vi "Set Visibility Of Queue List.vi"(8 "error in (no error)":errorcluster, 10 "Visible":bool, 11 "SongQueueActor in":refnum<class "SongQueueActor.lvclass">) -> (0 "error out":errorcluster, 3 "SongQueueActor out":refnum<class "SongQueueActor.lvclass">)   [LabVIEW 2015, in "SongQueueActor.lvlib" / "SongQueueActor.lvclass"]
uses:
  SongQueueActor.lvclass
  SongQueueActor.lvclass/SongQueueActor.ctl
  builds/xctls/Song Queue/Song Queue.lvlibp/app/xctls/SongQueue/Song Queue.xctl
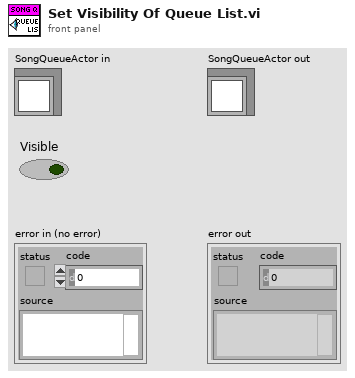
[diagram p1: front panel]
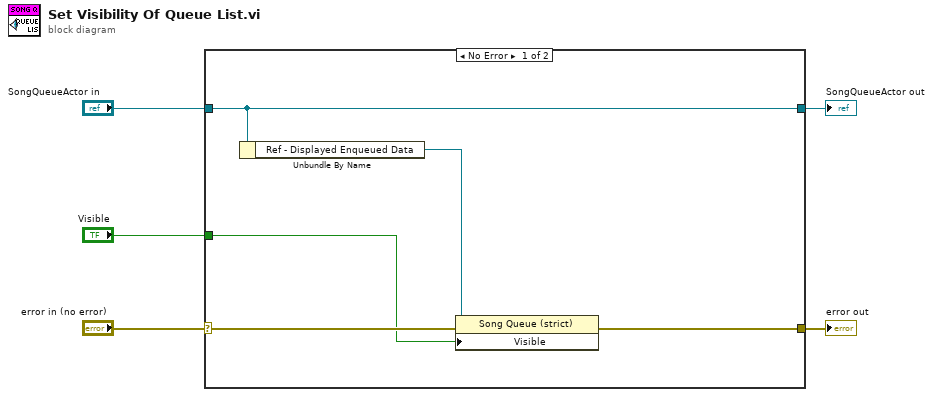
[diagram p0: block diagram]
diagram:
  n1 = case shown="No Error" "error in (no error)" {
    selector: "error in (no error)" -> [w9 w12]
    tunnel: [w7 w12] -> w4
    tunnel: [w10 w11] -> w2
    tunnel: "SongQueueActor in" -> [w10 w11]
    tunnel: "Visible" -> [w6 _]
    frame No Error {
      n2 = Unbundle By Name(w10) -> ("Ref - Displayed Enqueued Data"=w8:refnum<vi>)
      n3 = property class="Song Queue (strict)"(reference=w8, error in=w9, "Visible"=w6) -> (error out=w7:errorcluster)  [unwired: 1 out]
    }
    frame Error {
    }
  }
  "error out" <- w4
  "SongQueueActor out" <- w2
